vi "Read Config File.vi"(8 "error in (no error)":errorcluster) -> (0 "error out":errorcluster, 3 "Settings Out":T1)   [LabVIEW 2018, in "MWWL Verification.lvlib" / "MWWL Verification.lvclass"]
uses:
  MWWL Verification.lvclass
  Type Defs/ConfigSettings.ctl
  <vilib>/Utility/config.llb/Read Key (String).vi
  <vilib>/Utility/config.llb/NI_LVConfig.lvlib
  MWWL Verification.lvlib
panel:
  in  "Settings In":T1
  # "SM140"
  # "SM140"
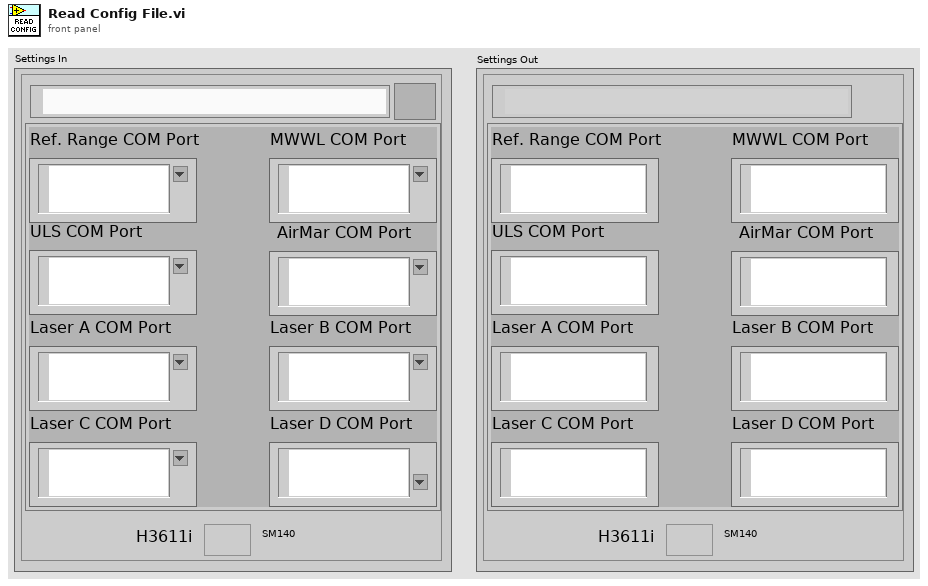
[diagram p1: front panel]
types:
  T1 = typedef "MWWL Verification.lvlib/ConfigSettings.ctl" = cluster{"Base Path":path, "DNL_Configuration Settings.Ports":cluster{"Ref. Range COM Port":refnum<visa-resource-name>, "MWWL COM Port":refnum<visa-resource-name>, "ULS COM Port":refnum<visa-resource-name>, "Laser A COM Port":refnum<visa-resource-name>, "Laser B COM Port":refnum<visa-resource-name>, "Laser C COM Port":refnum<visa-resource-name>, "Laser D COM Port":refnum<visa-resource-name>, "AirMar COM Port":refnum<visa-resource-name>}, "H3611i":bool}
  T2 = typedef "NI_LVConfig.lvlib/Config Data RefNum.ctl" = refnum<k1>
  T3 = cluster{"[0]":refnum<visa-resource-name>, "[1]":refnum<visa-resource-name>, "[2]":refnum<visa-resource-name>, "[3]":refnum<visa-resource-name>, "[4]":refnum<visa-resource-name>, "[5]":refnum<visa-resource-name>, "[6]":refnum<visa-resource-name>, "[7]":refnum<visa-resource-name>}
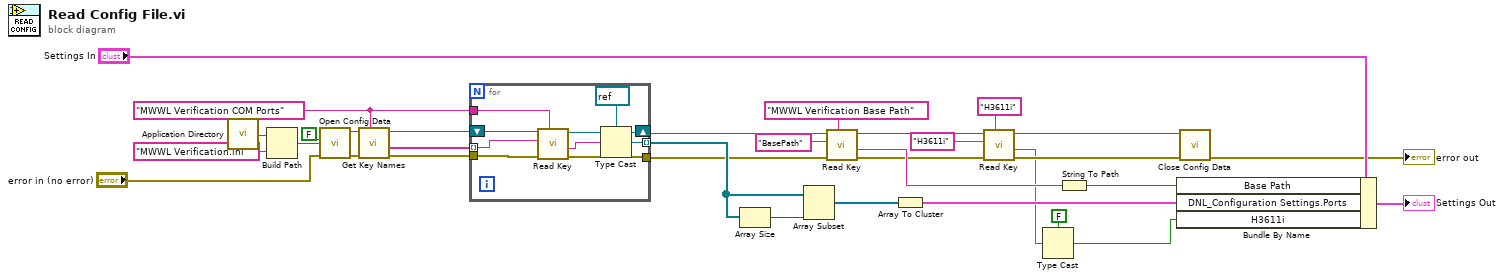
[diagram p0: block diagram]
diagram:
  w24 = "MWWL Verification COM Ports" ("section")
  n1 = call <vilib>:"Application Directory.vi"() -> ("Application Directory"=w32:path)
  n2 = Build Path(base path=w32, name or relative path="MWWL Verification.ini") -> (appended path=w30:path)
  n3 = call <vilib>:"Open Config Data.vi"("error in (no error)"="error in (no error)", "create file if necessary (T)"=FALSE, "configuration file path"=w30) -> ("error out"=w11:errorcluster, "refnum"=w27:T2)  [unwired: 6 in, 1 out]
  n4 = call <vilib>:"Get Key Names.vi"("section"=w24, "error in (no error)"=w11, "refnum"=w27) -> ("error out"=w26:errorcluster, "key names"=w25:string[], "refnum out"=w28:T2)  [unwired: 5 in, 1 out]
  n5 = for {
    tunnel: w26 -> [w40]
    tunnel: w25 -> [w42] mode=indexing
    tunnel: w24 -> [w39]
    tunnel: [w36] -> w23 mode=indexing
    shift-right: [w35] -> w18
    shift-left: w28 -> [w41]
    tunnel: [w34] -> w19
    n6 = call-poly <vilib>:"Read Key.vi"("section"=w39, "error in (no error)"=w40, "key"=w42, "refnum"=w41) -> ("error out"=w34:errorcluster, "value"=w38:string, "refnum out"=w35:T2)  [unwired: 4 in, 1 out]
    n7 = Type Cast(type=refnum<visa-resource-name> refnum ("DNL_Configuration Settings.Reference Range COM Port"), x=w38) -> (*(type *) &x=w36:refnum<visa-resource-name>)
  }
  n8 = Array Size(array=w23) -> (size(s)=w21:i32)
  n9 = Array Subset(array=w23, length=w21) -> (w22:refnum<visa-resource-name>[])  [unwired: 1 in]
  n10 = call-poly <vilib>:"Read Key.vi"("section"="MWWL Verification Base Path", "error in (no error)"=w19, "key"="BasePath" ("section"), "refnum"=w18) -> ("error out"=w5:errorcluster, "value"=w15:string, "refnum out"=w7:T2)  [unwired: 4 in, 1 out]
  n11 = Array To Cluster(array=w22) -> (cluster=w20:T3)
  n12 = call-poly <vilib>:"Read Key.vi"("section"="H3611i", "error in (no error)"=w5, "key"="H3611i" ("section"), "refnum"=w7) -> ("error out"=w4:errorcluster, "value"=w1:string, "refnum out"=w6:T2)  [unwired: 4 in, 1 out]
  n13 = Type Cast(type=FALSE ("H3611i"), x=w1) -> (*(type *) &x=w2:bool)
  n14 = String To Path(string=w15) -> (path=w14:path)
  n15 = Bundle By Name(cluster="Settings In", "Base Path"=w14, "DNL_Configuration Settings.Ports"=w20, "H3611i"=w2) -> (→"Settings Out":T1)
  n16 = call <vilib>:"Close Config Data.vi"("error in (no error)"=w4, "refnum"=w6) -> ("error out"=→"error out":errorcluster)  [unwired: 8 in, 1 out]
